vi "Create Frame Pattern Script.vi"(8 "error in (no error)":errorcluster, 10 "SPI_FRM_Config":T1 {"Addr" format="%x"; "Data" format="%x"}, 11 "SPI_Frame_WR in":refnum<class "SPI_Frame_WR.lvclass">) -> (0 "error out":errorcluster, 3 "SPI_Frame_WR out":refnum<class "SPI_Frame_WR.lvclass">)   [LabVIEW 2018, in "SPI_Frame_WR.lvclass"]
uses:
  SPI_Frame_WR.lvclass
  C:/P4 Workspace/PC Client/Solutions/5g_eap/HiSi/trunk/1.0/BML_Pattern_Gen_Refactor/SPI/SPI Frame Root/SPI_Frame_Root.lvclass
  Config Read SPI/SPI_FRM_Config.ctl
  Classes/Config_Read/RW_Option.ctl
  Config Read SPI/SPI_Mode.ctl
  SPI_Frame_WR.lvclass/SPI_Frame_WR.ctl
  SPI Frame Root/SPI_Frame_Root.lvclass/SPI_Frame_Root.ctl
  Classes/BML_Frame_Root/Special Frame.ctl
  SPI Frame Write/SPI_Frame_Write.lvclass
  SPI Frame Read Compare/SPI_Frame_Read_Compare.lvclass
  SPI_Frame_Read_Collect/SPI_Frame_Read_Collect.lvclass
  SPI Frame Root/SPI_Frame_Root.lvclass
  Classes/BML_Frame_Root/BML_Frame_Root.lvclass
  Classes/Config_Read/Config_Read_BML.lvclass
  Config Read SPI/Config_Read_SPI.lvclass
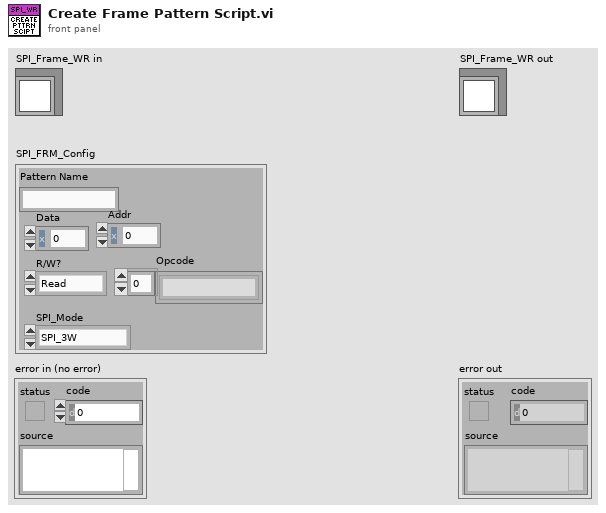
[diagram p1: front panel]
types:
  T1 = typedef "Config_Read_SPI.lvclass/SPI_FRM_Config.ctl" = cluster{"Pattern Name":string, "Data":u16, "Addr":u16, "R/W?":T2, "Opcode":string[], "SPI_Mode":T3}
  T2 = typedef "Config_Read_BML.lvclass/RW_Option.ctl" = enum16{"Read", "Write", "R/W"}
  T3 = typedef "Config_Read_SPI.lvclass/SPI_Mode.ctl" = enum16{"SPI_3W", "SPI_4W"}
  T4 = typedef "BML_Frame_Root.lvclass/Special Frame.ctl" = enum16{"Sync Header", "Protocol Header", "SW Trig", "SetID State", "Out SetID State", "SW Reset", "Wait", "SPI 4W FRM Start", "SPI 4W Wait", "SPI 4W FRM End", "SPI 4W Write Cmd", "SPI RD Collect Cmd", "SPI RD Value Cmd", "SPI 3W FRM Start", "SPI 3W Write Cmd", "SPI 3W FRM End", "SPI 3W Wait", "SPI 3W RD Cmd"}
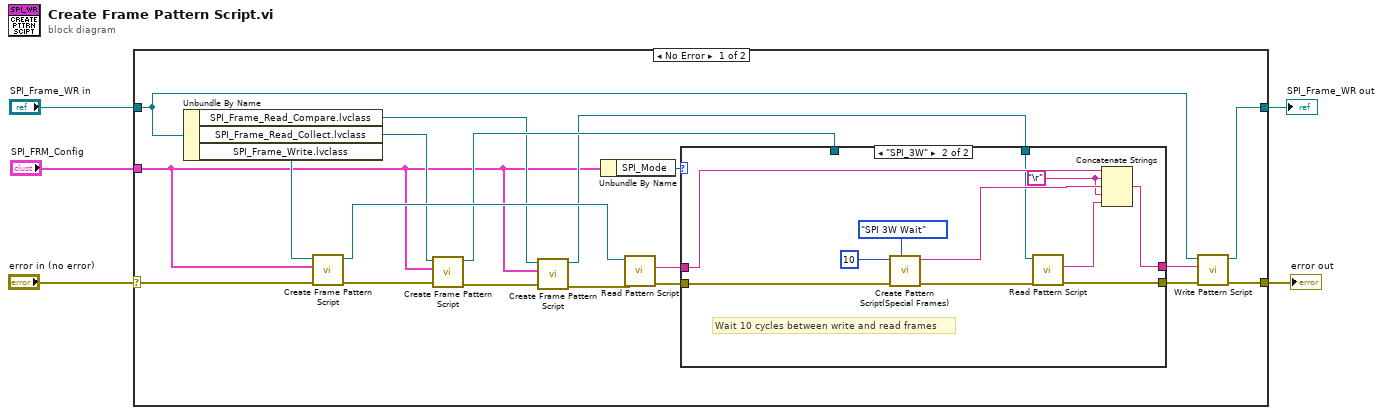
[diagram p0: block diagram]
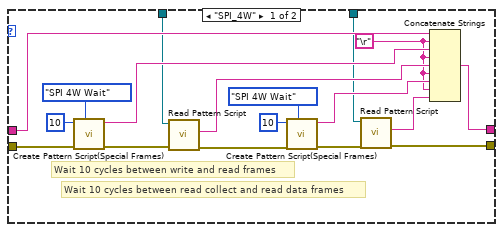
[diagram p2: hidden frame]
diagram:
  n1 = case shown="No Error" "error in (no error)" {
    selector: "error in (no error)" -> [w17 w55]
    tunnel: "SPI_Frame_WR in" -> [w20 w54]
    tunnel: [w21 w55] -> w3
    tunnel: [w19 w54] -> w2
    tunnel: "SPI_FRM_Config" -> [w7 _]
    frame No Error {
      n2 = Unbundle By Name(w20) -> ("SPI_Frame_Read_Compare.lvclass"=w11:refnum<class "SPI_Frame_Read_Compare.lvclass">, "SPI_Frame_Read_Collect.lvclass"=w13:refnum<class "SPI_Frame_Read_Collect.lvclass">, "SPI_Frame_Write.lvclass"=w16:refnum<class "SPI_Frame_Write.lvclass">)
      n3 = call-dynamic "Create Frame Pattern Script.vi"("error in (no error)"=w17, "SPI_FRM_Config"=w7, "SPI_Frame_Write in"=w16) -> ("error out"=w14:errorcluster, "SPI_Frame_Write out"=w15:refnum<class "SPI_Frame_Write.lvclass">)  [unwired: 7 in]
      n4 = call-dynamic "Create Frame Pattern Script.vi"("error in (no error)"=w14, "SPI_FRM_Config"=w7, "SPI_Frame_Read_Collect in"=w13) -> ("error out"=w10:errorcluster, "SPI_Frame_Read_Collect out"=w12:refnum<class "SPI_Frame_Read_Collect.lvclass">)  [unwired: 7 in]
      n5 = call-dynamic "Create Frame Pattern Script.vi"("error in (no error)"=w10, "SPI_FRM_Config"=w7, "SPI_Frame_Read_Compare in"=w11) -> ("error out"=w9:errorcluster, "SPI_Frame_Read_Compare out"=w8:refnum<class "SPI_Frame_Read_Compare.lvclass">)  [unwired: 7 in]
      n6 = Unbundle By Name(w7) -> ("SPI_Mode"=w6:T3)
      n7 = call "Read Pattern Script.vi"("error in (no error)"=w9, "SPI_Frame_Root in"=w15) -> ("error out"=w24:errorcluster, "Pattern Script"=w23:string)  [unwired: 7 in, 1 out]
      n8 = case shown="\"SPI_3W\"" w6 {
        tunnel: w24 -> [w42 w53]
        tunnel: w23 -> [w36 w51]
        tunnel: [w30 w48] -> w22
        tunnel: [w29 w47] -> w18
        tunnel: w12 -> [w28 _]
        tunnel: w8 -> [w27 w46]
        frame "SPI_4W" {
          w32 = "\r"
          # "Wait 10 cycles between read collect and read data frames"
          # "Wait 10 cycles between write and read frames"
          n9 = call "Create Pattern Script(Special Frames).vi"("Special Frame Type"=Special_Frame."SPI 4W Wait", "error in (no error)"=w42, "Num of Timeset"=u32 10) -> ("error out"=w41:errorcluster, "string out"=w35:string)  [unwired: 7 in]
          n10 = call "Read Pattern Script.vi"("error in (no error)"=w41, "SPI_Frame_Root in"=w28) -> ("error out"=w38:errorcluster, "Pattern Script"=w34:string)  [unwired: 7 in, 1 out]
          n11 = call "Create Pattern Script(Special Frames).vi"("Special Frame Type"=Special_Frame."SPI 4W Wait", "error in (no error)"=w38, "Num of Timeset"=u32 10) -> ("error out"=w39:errorcluster, "string out"=w33:string)  [unwired: 7 in]
          n12 = call "Read Pattern Script.vi"("error in (no error)"=w39, "SPI_Frame_Root in"=w27) -> ("error out"=w30:errorcluster, "Pattern Script"=w31:string)  [unwired: 7 in, 1 out]
          n13 = Concatenate Strings(w36, w32, w35, w32, w34, w32, w33, w32, w31) -> (w29:string)
        }
        frame "SPI_3W" {
          w49 = "\r"
          # "Wait 10 cycles between write and read frames"
          n14 = call "Create Pattern Script(Special Frames).vi"("Special Frame Type"=Special_Frame."SPI 3W Wait", "error in (no error)"=w53, "Num of Timeset"=u32 10) -> ("error out"=w44:errorcluster, "string out"=w50:string)  [unwired: 7 in]
          n15 = call "Read Pattern Script.vi"("error in (no error)"=w44, "SPI_Frame_Root in"=w46) -> ("error out"=w48:errorcluster, "Pattern Script"=w43:string)  [unwired: 7 in, 1 out]
          n16 = Concatenate Strings(w51, w49, w50, w49, w43) -> (w47:string)
        }
      }
      n17 = call "Write Pattern Script.vi"("error in (no error)"=w22, "Pattern Script"=w18, "SPI_Frame_Root in"=w20) -> ("error out"=w21:errorcluster, "SPI_Frame_Root out"=w19:refnum<class "SPI_Frame_WR.lvclass">)  [unwired: 7 in]
    }
    frame Error {
    }
  }
  "error out" <- w3
  "SPI_Frame_WR out" <- w2
